vi "Nav Testing 1.vi"() -> ()   [LabVIEW 2015]
panel:
  out "Right Duty Cycle":dbl=0.5
  out "Left Duty Cycle":dbl=0.5
  in  "Dest Y":dbl
  in  "Dest X":dbl
  in  "Start Y":dbl
  in  "Start X":dbl
  # "Moves robot between two specified points.\nNo localization data required.\n\nImplements basic motor control."
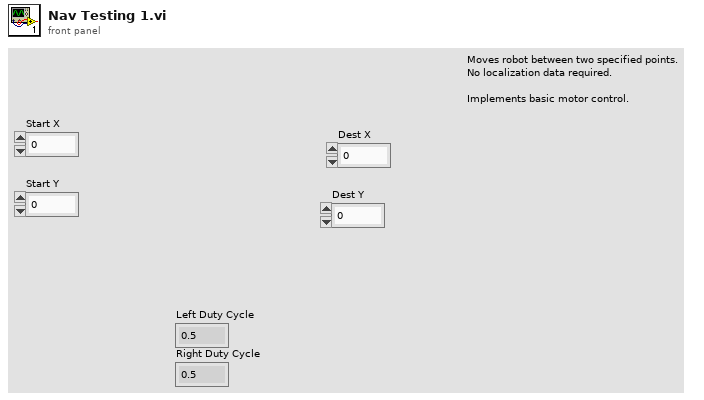
[diagram p1: front panel]
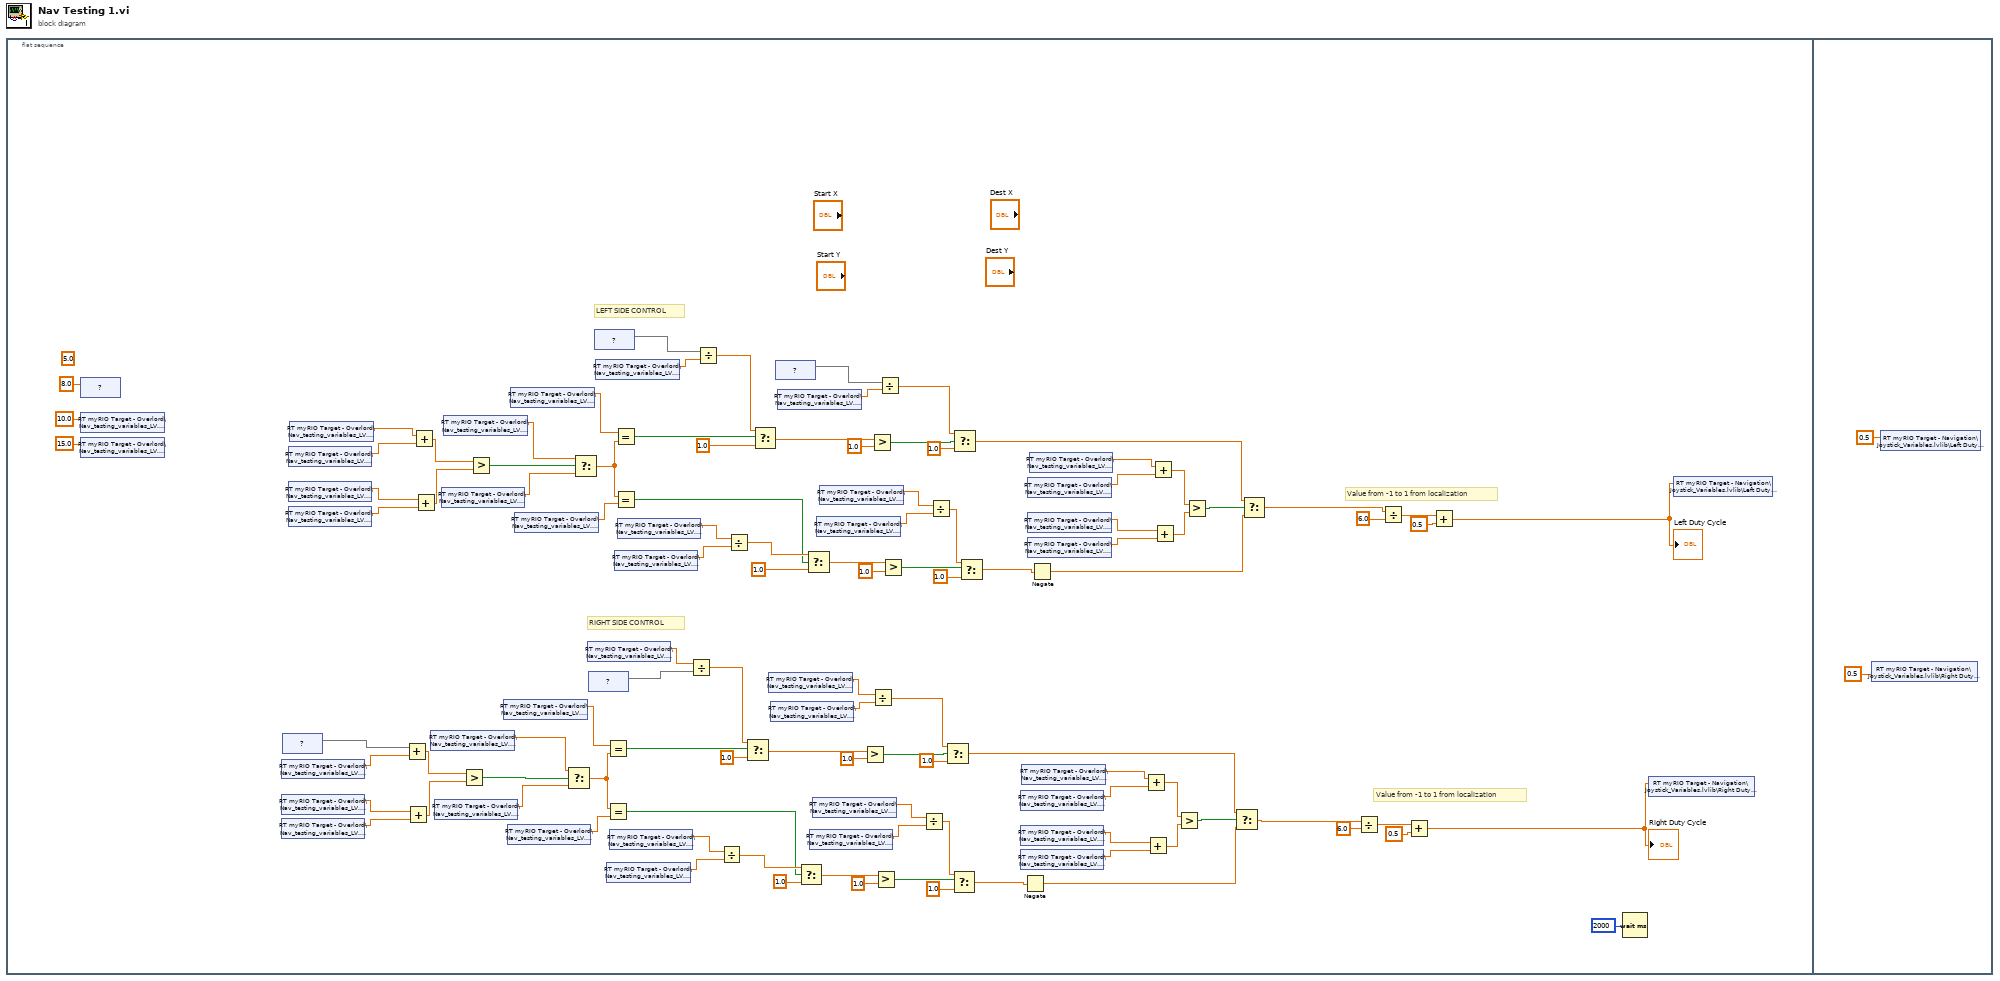
[diagram p0: block diagram]
diagram:
  n1 = flat-sequence {
    frame #0 {
      (unwired) 5.0 ("cornerDist1")
      # "RIGHT SIDE CONTROL"
      # "LEFT SIDE CONTROL"
      # "Value from -1 to 1 from localization"
      # "Value from -1 to 1 from localization"
      n2 = shared-variable "?"(8.0 ("cornerDist2")) -> ()  [unwired: 1 in, 1 out]
      n3 = shared-variable "RT myRIO Target - Overlord\\Nav_testing_variables_LV.lvlib\\cornerDist3"(10.0 ("cornerDist3")) -> ()  [unwired: 1 in, 1 out]
      n4 = shared-variable "RT myRIO Target - Overlord\\Nav_testing_variables_LV.lvlib\\cornerDist4"(15.0 ("cornerDist4")) -> ()  [unwired: 1 in, 1 out]
      n5 = shared-variable "RT myRIO Target - Overlord\\Nav_testing_variables_LV.lvlib\\cornerDist2"() -> (w47:dbl)  [unwired: 1 in, 1 out]
      n6 = shared-variable "RT myRIO Target - Overlord\\Nav_testing_variables_LV.lvlib\\cornerDist3"() -> (w50:dbl)  [unwired: 1 in, 1 out]
      n7 = shared-variable "RT myRIO Target - Overlord\\Nav_testing_variables_LV.lvlib\\cornerDist4"() -> (w49:dbl)  [unwired: 1 in, 1 out]
      n8 = shared-variable "?"() -> (w48)  [unwired: 1 in, 1 out]
      n9 = shared-variable "RT myRIO Target - Overlord\\Nav_testing_variables_LV.lvlib\\cornerDist2"() -> (w92:dbl)  [unwired: 1 in, 1 out]
      n10 = shared-variable "RT myRIO Target - Overlord\\Nav_testing_variables_LV.lvlib\\cornerDist3"() -> (w95:dbl)  [unwired: 1 in, 1 out]
      n11 = shared-variable "RT myRIO Target - Overlord\\Nav_testing_variables_LV.lvlib\\cornerDist4"() -> (w94:dbl)  [unwired: 1 in, 1 out]
      n12 = shared-variable "RT myRIO Target - Overlord\\Nav_testing_variables_LV.lvlib\\cornerDist1"() -> (w93:dbl)  [unwired: 1 in, 1 out]
      n13 = Add(x=w48, y=w47) -> (x+y=w53:dbl)
      n14 = Add(x=w50, y=w49) -> (x+y=w52:dbl)
      n15 = Add(x=w93, y=w92) -> (x+y=w98:dbl)
      n16 = Add(x=w95, y=w94) -> (x+y=w97:dbl)
      n17 = shared-variable "RT myRIO Target - Overlord\\Nav_testing_variables_LV.lvlib\\cornerDist2"() -> (w10:dbl)  [unwired: 1 in, 1 out]
      n18 = shared-variable "RT myRIO Target - Overlord\\Nav_testing_variables_LV.lvlib\\cornerDist4"() -> (w46:dbl)  [unwired: 1 in, 1 out]
      n19 = shared-variable "RT myRIO Target - Overlord\\Nav_testing_variables_LV.lvlib\\cornerDist3"() -> (w91:dbl)  [unwired: 1 in, 1 out]
      n20 = shared-variable "RT myRIO Target - Overlord\\Nav_testing_variables_LV.lvlib\\cornerDist1"() -> (w90:dbl)  [unwired: 1 in, 1 out]
      n21 = Greater?(x=w53, y=w52) -> (0:w51:bool)
      n22 = Greater?(x=w98, y=w97) -> (0:w96:bool)
      n23 = shared-variable "RT myRIO Target - Overlord\\Nav_testing_variables_LV.lvlib\\cornerDist1"() -> (w45:dbl)  [unwired: 1 in, 1 out]
      n24 = shared-variable "RT myRIO Target - Overlord\\Nav_testing_variables_LV.lvlib\\cornerDist3"() -> (w43:dbl)  [unwired: 1 in, 1 out]
      n25 = shared-variable "RT myRIO Target - Overlord\\Nav_testing_variables_LV.lvlib\\cornerDist1"() -> (w89:dbl)  [unwired: 1 in, 1 out]
      n26 = shared-variable "RT myRIO Target - Overlord\\Nav_testing_variables_LV.lvlib\\cornerDist3"() -> (w87:dbl)  [unwired: 1 in, 1 out]
      n27 = Select(t=w10, s=w51, f=w46) -> (s? t:f=w44:dbl)
      n28 = Select(t=w90, s=w96, f=w91) -> (s? t:f=w88:dbl)
      n29 = shared-variable "RT myRIO Target - Overlord\\Nav_testing_variables_LV.lvlib\\cornerDist2"() -> (w41:dbl)  [unwired: 1 in, 1 out]
      n30 = shared-variable "?"() -> (w42)  [unwired: 1 in, 1 out]
      n31 = shared-variable "?"() -> (w85)  [unwired: 1 in, 1 out]
      n32 = shared-variable "RT myRIO Target - Overlord\\Nav_testing_variables_LV.lvlib\\cornerDist2"() -> (w86:dbl)  [unwired: 1 in, 1 out]
      n33 = Equal?(x=w45, y=w44) -> (x = y?=w40:bool)
      n34 = Equal?(x=w44, y=w43) -> (x = y?=w35:bool)
      n35 = shared-variable "RT myRIO Target - Overlord\\Nav_testing_variables_LV.lvlib\\cornerDist3"() -> (w37:dbl)  [unwired: 1 in, 1 out]
      n36 = shared-variable "RT myRIO Target - Overlord\\Nav_testing_variables_LV.lvlib\\cornerDist4"() -> (w38:dbl)  [unwired: 1 in, 1 out]
      n37 = Equal?(x=w89, y=w88) -> (x = y?=w84:bool)
      n38 = Equal?(x=w88, y=w87) -> (x = y?=w79:bool)
      n39 = shared-variable "RT myRIO Target - Overlord\\Nav_testing_variables_LV.lvlib\\cornerDist4"() -> (w81:dbl)  [unwired: 1 in, 1 out]
      n40 = shared-variable "RT myRIO Target - Overlord\\Nav_testing_variables_LV.lvlib\\cornerDist3"() -> (w82:dbl)  [unwired: 1 in, 1 out]
      n41 = Divide(x=w41, y=w42) -> (x/y=w39:dbl)
      n42 = Divide(x=w85, y=w86) -> (x/y=w83:dbl)
      n43 = Divide(x=w38, y=w37) -> (x/y=w36:dbl)
      n44 = Divide(x=w82, y=w81) -> (x/y=w80:dbl)
      n45 = Select(t=w39, s=w40, f=1.0) -> (s? t:f=w27:dbl)
      n46 = Select(t=w83, s=w84, f=1.0) -> (s? t:f=w71:dbl)
      n47 = shared-variable "RT myRIO Target - Overlord\\Nav_testing_variables_LV.lvlib\\cornerDist2"() -> (w22:dbl)  [unwired: 1 in, 1 out]
      n48 = shared-variable "RT myRIO Target - Overlord\\Nav_testing_variables_LV.lvlib\\cornerDist1"() -> (w23:dbl)  [unwired: 1 in, 1 out]
      n49 = shared-variable "?"() -> (w66)  [unwired: 1 in, 1 out]
      n50 = shared-variable "RT myRIO Target - Overlord\\Nav_testing_variables_LV.lvlib\\cornerDist2"() -> (w67:dbl)  [unwired: 1 in, 1 out]
      n51 = Select(t=w36, s=w35, f=1.0) -> (s? t:f=w34:dbl)
      n52 = Select(t=w80, s=w79, f=1.0) -> (s? t:f=w78:dbl)
      n53 = shared-variable "RT myRIO Target - Overlord\\Nav_testing_variables_LV.lvlib\\cornerDist3"() -> (w31:dbl)  [unwired: 1 in, 1 out]
      n54 = shared-variable "RT myRIO Target - Overlord\\Nav_testing_variables_LV.lvlib\\cornerDist4"() -> (w32:dbl)  [unwired: 1 in, 1 out]
      n55 = shared-variable "RT myRIO Target - Overlord\\Nav_testing_variables_LV.lvlib\\cornerDist4"() -> (w75:dbl)  [unwired: 1 in, 1 out]
      n56 = shared-variable "RT myRIO Target - Overlord\\Nav_testing_variables_LV.lvlib\\cornerDist3"() -> (w76:dbl)  [unwired: 1 in, 1 out]
      n57 = Greater?(x=w27, y=1.0) -> (0:w25:bool)
      n58 = Greater?(x=w71, y=1.0) -> (0:w69:bool)
      n59 = Divide(x=w22, y=w23) -> (x/y=w21:dbl)
      n60 = Greater?(x=w34, y=1.0) -> (0:w30:bool)
      n61 = Divide(x=w66, y=w67) -> (x/y=w65:dbl)
      n62 = Greater?(x=w78, y=1.0) -> (0:w74:bool)
      n63 = Divide(x=w32, y=w31) -> (x/y=w29:dbl)
      n64 = Divide(x=w76, y=w75) -> (x/y=w73:dbl)
      n65 = Select(t=w21, s=w25, f=1.0) -> (s? t:f=w14:dbl)
      n66 = Select(t=w29, s=w30, f=1.0) -> (s? t:f=w12:dbl)
      n67 = Select(t=w65, s=w69, f=1.0) -> (s? t:f=w58:dbl)
      n68 = Select(t=w73, s=w74, f=1.0) -> (s? t:f=w55:dbl)
      n69 = shared-variable "RT myRIO Target - Overlord\\Nav_testing_variables_LV.lvlib\\cornerDist2"() -> (w17:dbl)  [unwired: 1 in, 1 out]
      n70 = shared-variable "RT myRIO Target - Overlord\\Nav_testing_variables_LV.lvlib\\cornerDist3"() -> (w20:dbl)  [unwired: 1 in, 1 out]
      n71 = shared-variable "RT myRIO Target - Overlord\\Nav_testing_variables_LV.lvlib\\cornerDist4"() -> (w19:dbl)  [unwired: 1 in, 1 out]
      n72 = shared-variable "RT myRIO Target - Overlord\\Nav_testing_variables_LV.lvlib\\cornerDist1"() -> (w18:dbl)  [unwired: 1 in, 1 out]
      n73 = Negate(x=w12) -> (-x=w11:dbl)
      n74 = shared-variable "RT myRIO Target - Overlord\\Nav_testing_variables_LV.lvlib\\cornerDist2"() -> (w61:dbl)  [unwired: 1 in, 1 out]
      n75 = shared-variable "RT myRIO Target - Overlord\\Nav_testing_variables_LV.lvlib\\cornerDist3"() -> (w64:dbl)  [unwired: 1 in, 1 out]
      n76 = shared-variable "RT myRIO Target - Overlord\\Nav_testing_variables_LV.lvlib\\cornerDist4"() -> (w63:dbl)  [unwired: 1 in, 1 out]
      n77 = shared-variable "RT myRIO Target - Overlord\\Nav_testing_variables_LV.lvlib\\cornerDist1"() -> (w62:dbl)  [unwired: 1 in, 1 out]
      n78 = Negate(x=w55) -> (-x=w54:dbl)
      n79 = Add(x=w18, y=w17) -> (x+y=w16:dbl)
      n80 = Add(x=w20, y=w19) -> (x+y=w15:dbl)
      n81 = Add(x=w62, y=w61) -> (x+y=w60:dbl)
      n82 = Add(x=w64, y=w63) -> (x+y=w59:dbl)
      n83 = Greater?(x=w16, y=w15) -> (0:w13:bool)
      n84 = Greater?(x=w60, y=w59) -> (0:w57:bool)
      n85 = Select(t=w14, s=w13, f=w11) -> (s? t:f=w9:dbl)
      n86 = Select(t=w58, s=w57, f=w54) -> (s? t:f=w56:dbl)
      n87 = Divide(x=w9, y=6.0) -> (x/y=w105:dbl)
      n88 = Divide(x=w56, y=6.0) -> (x/y=w101:dbl)
      n89 = Add(x=w105, y=0.5) -> (x+y=w103:dbl)
      "Right Duty Cycle" <- w103
      n90 = Add(x=w101, y=0.5) -> (x+y=w99:dbl)
      "Left Duty Cycle" <- w99
      n91 = Wait (ms)(milliseconds to wait=u32 2000) -> ()  [unwired: 1 out]
      n92 = shared-variable "RT myRIO Target - Navigation\\Joystick_Variables.lvlib\\Right Duty Cycle"(w103) -> ()  [unwired: 1 in, 1 out]
      n93 = shared-variable "RT myRIO Target - Navigation\\Joystick_Variables.lvlib\\Left Duty Cycle"(w99) -> ()  [unwired: 1 in, 1 out]
    }
    frame #1 {
      n94 = shared-variable "RT myRIO Target - Navigation\\Joystick_Variables.lvlib\\Right Duty Cycle"(0.5 ("Right Duty Cycle 2")) -> ()  [unwired: 1 in, 1 out]
      n95 = shared-variable "RT myRIO Target - Navigation\\Joystick_Variables.lvlib\\Left Duty Cycle"(0.5 ("Left Duty Cycle")) -> ()  [unwired: 1 in, 1 out]
    }
  }
